vi "Main.vi"(10 "Sub Panel":refnum<vi>, 11 "Module Admin":refnum<class "Delacor_lib_QMH_Module Admin.lvclass">) -> ()   [LabVIEW 2020, in "Acquisition.lvlib"]
doc: "This template is based off of the Queued Message Handler design pattern and the Queued Message Handler project template that ships with LabVIEW.\n\nThe main difference is that the queue is private to this module and communication between modules is performed via Broadcast and Request events.\n\nRequest events are wrapped in public API methods and are handled in the Event Handling Loop (EHL) of this VI. Any module can register for Broadcast events sent by this module. The EHL generates messages based on user interface actions.\n\nThe Message Handling Loop (MHL) processes messages generated by the EHL, or by other messages. The messages are string values, so new messages can be added easily to the Message Cases case structure in the MHL. Each message cluster can also provide an optional value for Message Data, which is a variant that can be converted to whatever message-specific data is required.\n_____\nBased on Delacor QMH Project Template 5.0.0.82."
uses:
  Acquisition.lvlib
  <vilib>/Delacor/Delacor QMH/Libraries/Module Admin_class/Delacor_lib_QMH_Module Admin.lvclass
  Module Data--cluster.ctl
  Stop Helper Loop Argument--cluster.ctl
  Stop Argument--cluster.ctl
  <vilib>/Delacor/Delacor QMH/Libraries/Message Queue_class/Delacor_lib_QMH_Message Queue.lvclass/Delacor_lib_QMH_Message Queue.ctl
  <vilib>/Delacor/Delacor QMH/Libraries/Module Admin_class/Delacor_lib_QMH_Module Admin.lvclass/Delacor_lib_QMH_Module Admin.ctl
  <vilib>/Utility/miscctls.llb/LVPointTypeDef.ctl
  <vilib>/Delacor/Delacor QMH/Libraries/Message Queue_class/Delacor_lib_QMH_Enqueue Message (Single).vi
  <vilib>/Delacor/Delacor QMH/Libraries/Module Admin_class/Delacor_lib_QMH_Get External Launch.vi
  <vilib>/Utility/error.llb/Error Cluster From Error Code.vi
  <vilib>/ErrorRing/Error Ring.xnode
  <vilib>/Delacor/Delacor QMH/Libraries/Message Queue_class/Delacor_lib_QMH_Message Queue.lvclass
  <vilib>/measure/NI_MABase.lvlib
panel:
  out "Waveform Graph":waveform(dbl)(graph)
  out "error out":errorcluster
  out "Status":string
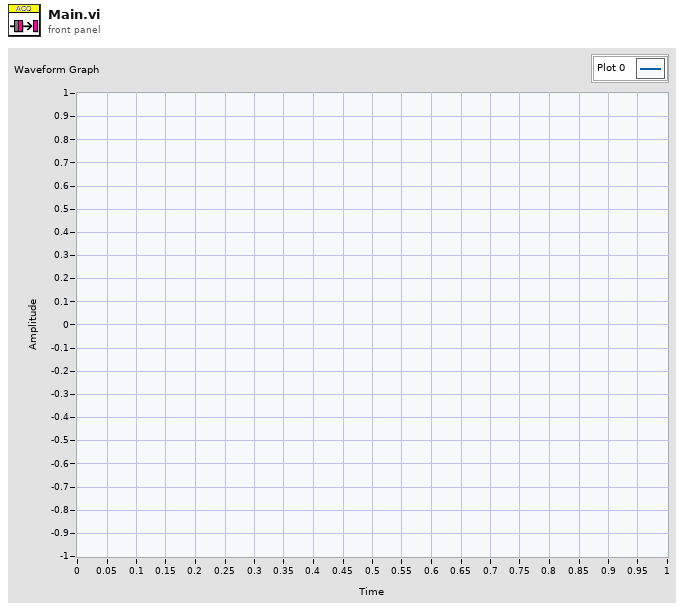
[diagram p1: front panel]
types:
  T1 = typedef "Acquisition.lvlib/Request Events--cluster.ctl" = cluster{"Stop Module":refnum<user-event>, "Show Panel":refnum<user-event>, "Hide Panel":refnum<user-event>, "Get Module Execution Status":refnum<user-event>, "Show Diagram":refnum<user-event>, "Start Helper Loop":refnum<user-event>, "Stop Helper Loop":refnum<user-event>, "Set Acquisition Config":refnum<user-event>}
  T2 = typedef "Acquisition.lvlib/Module Data--cluster.ctl" = cluster{"Status":string}
  T3 = typedef "Acquisition.lvlib/Stop Helper Loop Argument--cluster.ctl" = cluster{"Boolean":bool}
  T4 = enum32{"invalid lock state", "Not Locked", "Locked (No Password)", "Password-protected"}
  T5 = typedef "Acquisition.lvlib/Stop Argument--cluster.ctl" = cluster{"Origin":string, "Exit via Stop Module Req?":bool, "Wait for Module to stop?":bool}
  T6 = typedef "LVPointTypeDef.ctl" = cluster{"Horizontal":i16, "Vertical":i16}
  T7 = enum32{"Invalid", "Standard", "Closed", "Hidden", "Minimized", "Maximized"}
  T8 = enum16{"Sine Wave", "Triangle Wave", "Square Wave", "Sawtooth Wave"}
  T9 = cluster{"sampling info":cluster{"Fs":dbl, "#s":dbl}, "square wave duty cycle (%)":dbl, "frequency":dbl, "amplitude":dbl, "phase":dbl, "signal type":enum16{"Sine Wave", "Triangle Wave", "Square Wave", "Sawtooth Wave"}}
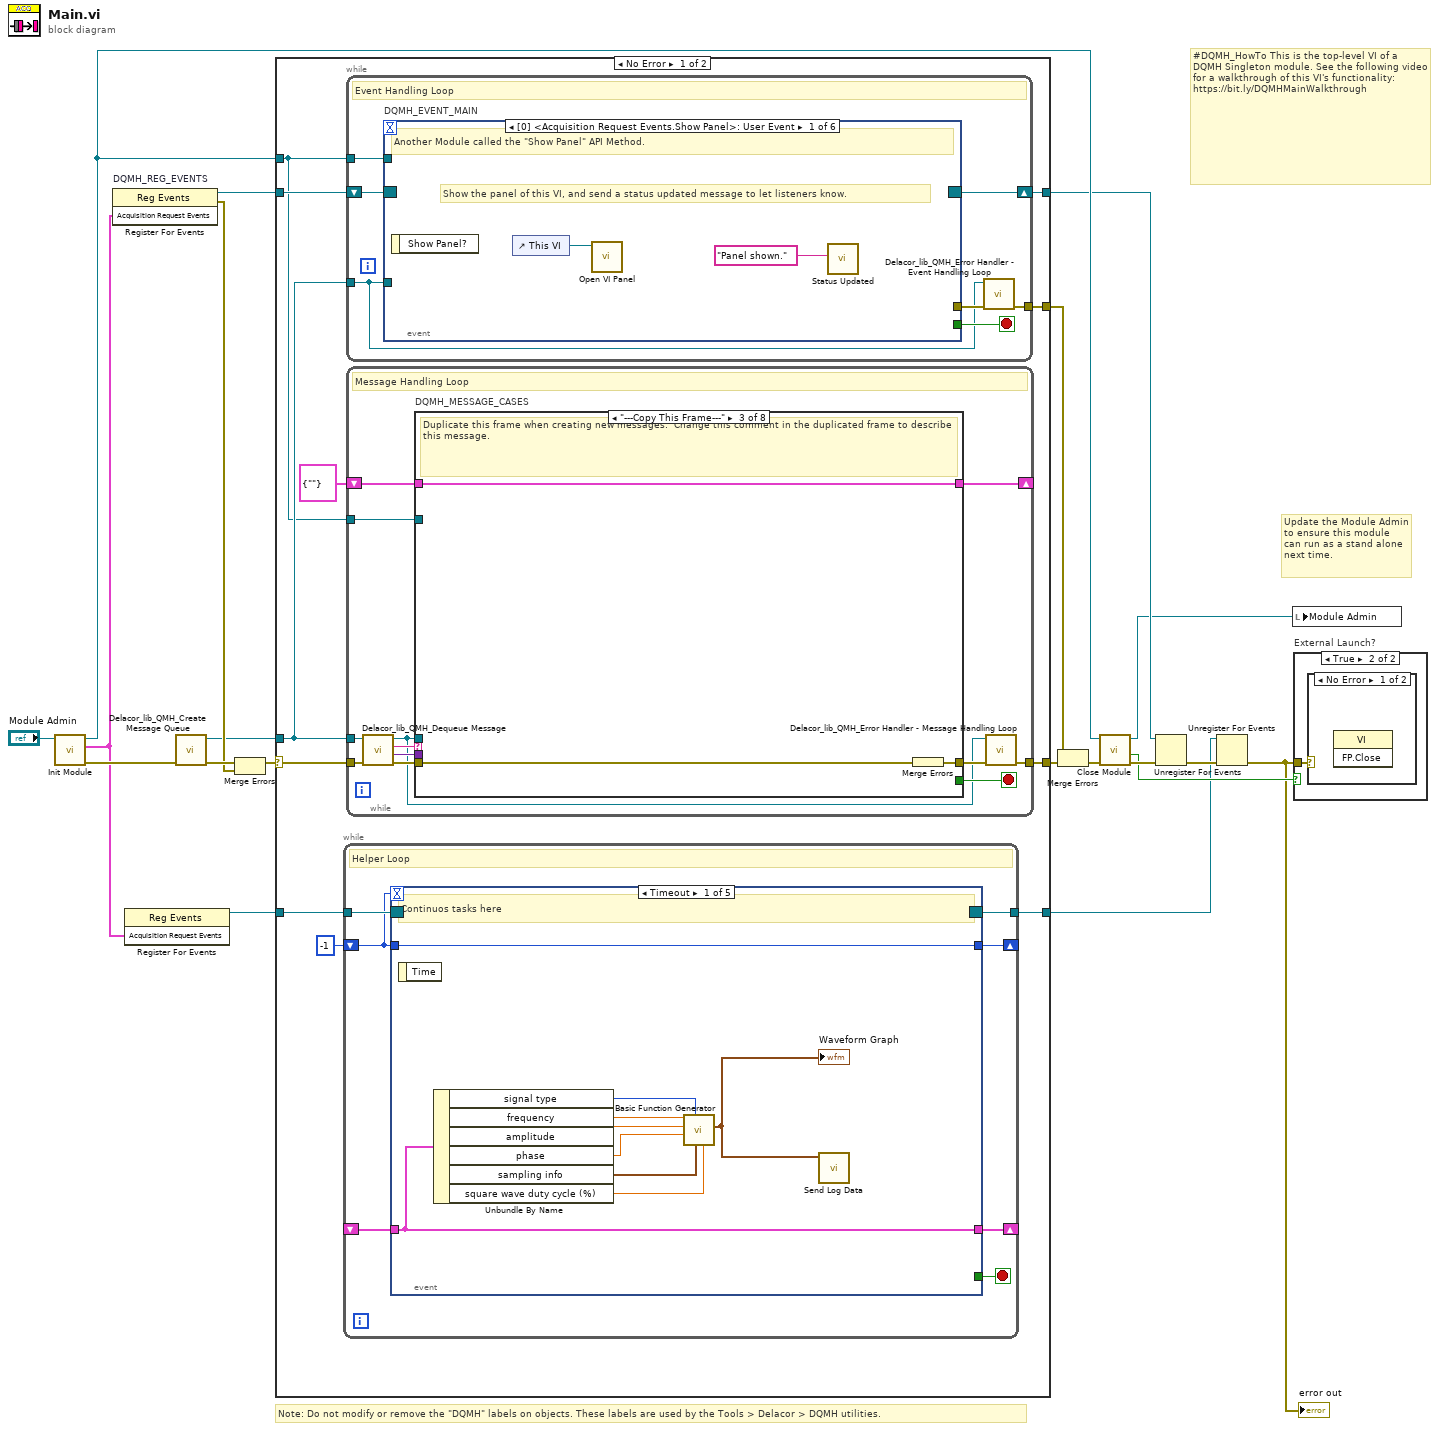
[diagram p0: block diagram]
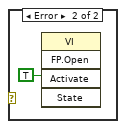
[diagram p3: hidden frame]
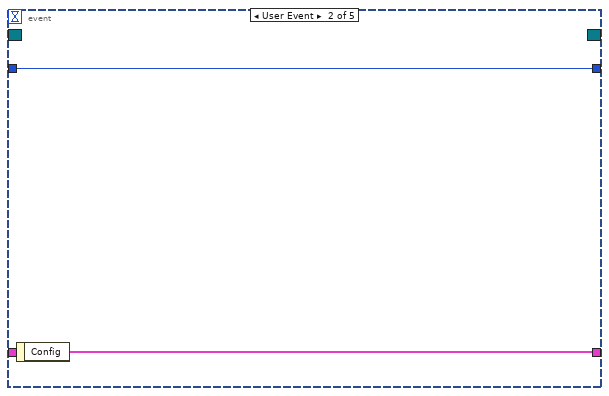
[diagram p4: hidden frame]
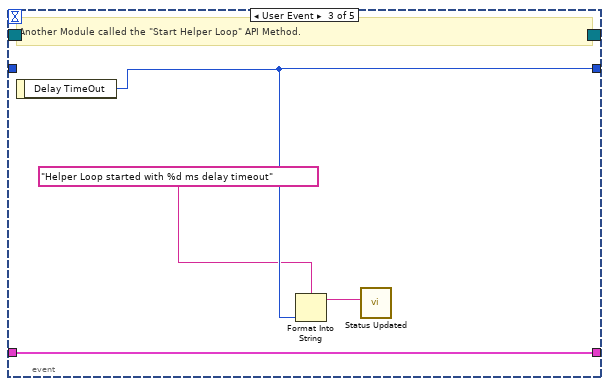
[diagram p5: hidden frame]
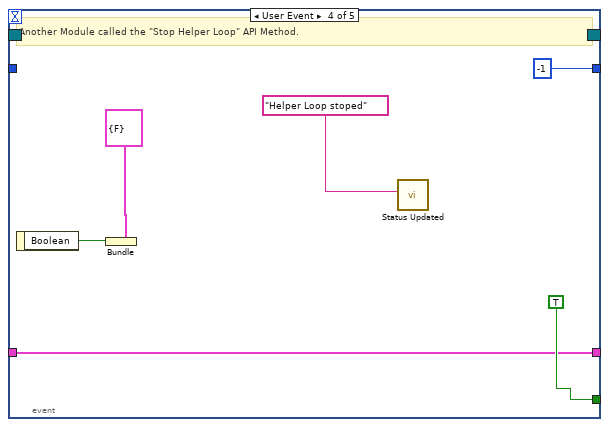
[diagram p6: hidden frame]
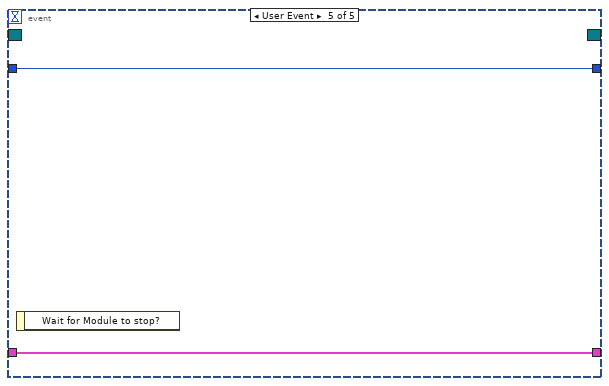
[diagram p7: hidden frame]
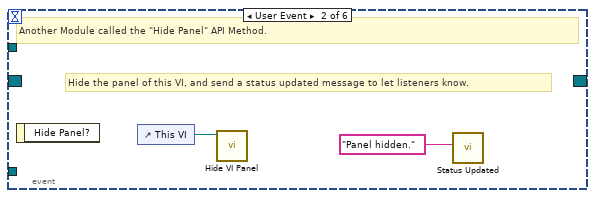
[diagram p8: hidden frame]
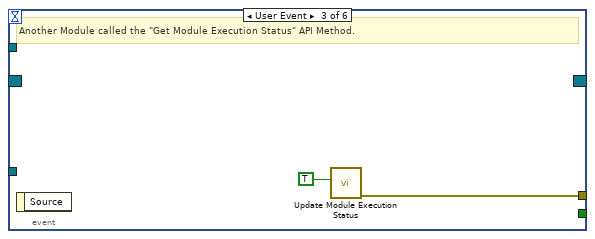
[diagram p9: hidden frame]
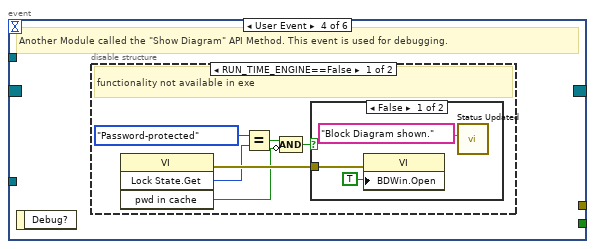
[diagram p10: hidden frame]
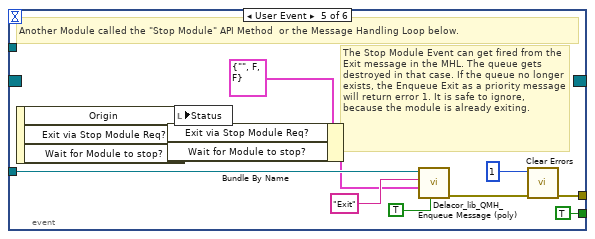
[diagram p13: hidden frame]
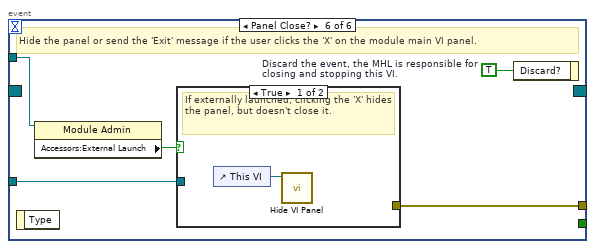
[diagram p14: hidden frame]
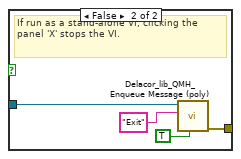
[diagram p15: hidden frame]
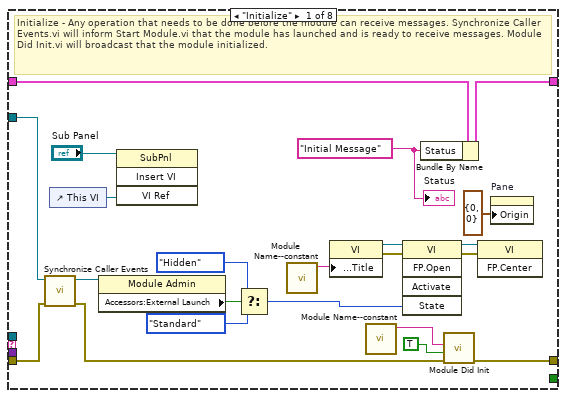
[diagram p16: hidden frame]
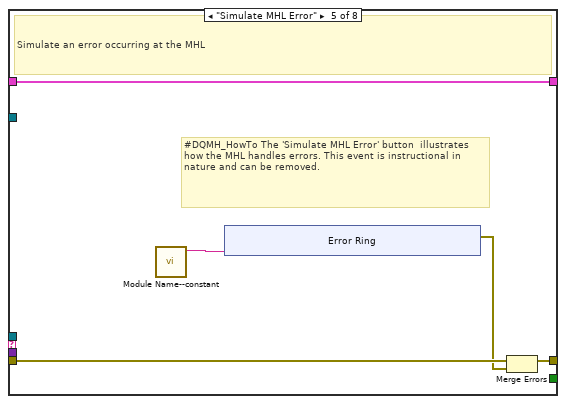
[diagram p19: hidden frame]
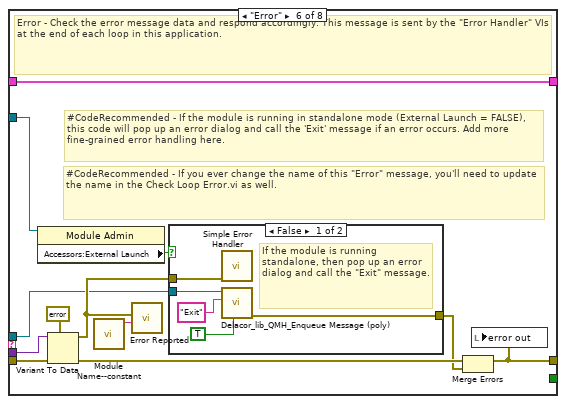
[diagram p20: hidden frame]
diagram:
  # "#DQMH_HowTo This is the top-level VI of a DQMH Singleton module. See the following video for a walkthrough of this VI's functionality: https://bit.ly/DQMHMainWalkthrough"
  # "Note: Do not modify or remove the \"DQMH\" labels on objects. These labels are used by the Tools > Delacor > DQMH utilities."
  # "Update the Module Admin to ensure this module can run as a stand alone next time."
  n1 = call "Init Module.vi"("Singleton Module Admin in"="Module Admin") -> ("error out"=w19:errorcluster, "Acquisition Request Events"=w3:T1, "Singleton Module Admin out"=w11:refnum<class "Delacor_lib_QMH_Module Admin.lvclass">)  [unwired: 8 in]
  n2 = register-events "DQMH_REG_EVENTS"(w3) -> (reference out=w9:refnum<event-registration>, error out=w12:errorcluster)  [unwired: 2 in]
  n3 = register-events(w3) -> (reference out=w4:refnum<event-registration>)  [unwired: 2 in, 1 out]
  n4 = call <vilib>:"Delacor_lib_QMH_Create Message Queue.vi"("error in (no error)"=w19) -> ("error out"=w14:errorcluster, "Message Queue"=w8:refnum<class "Delacor_lib_QMH_Message Queue.lvclass">)  [unwired: 9 in]
  n5 = Merge Errors(w14, w12) -> (w13:errorcluster)
  n6 = case shown="No Error" w13 {
    selector: w13 -> [w29 w207]
    tunnel: [w31 w206] -> w20
    tunnel: [w28 w212] -> w10
    tunnel: w9 -> [w26 w212]
    tunnel: w8 -> [w25 w205]
    tunnel: [w30 _] -> w17
    tunnel: w11 -> [w24 w208]
    tunnel: w4 -> [w23 _]
    tunnel: [w22 _] -> w1
    frame No Error {
      n7 = while {
        tunnel: w23 -> [w38]
        tunnel: [w37] -> w22
        shift-right: [w36] -> _
        shift-left: -1 -> [w35]
        shift-right: [w33] -> _
        shift-left: _ -> [w32]
        stop <- w34 stop-if-true
        # "Helper Loop"
        n8 = event shown="[0] Timeout" {
          selector: w38 -> [_ _ _ _ _]
          dyn-events: [_ _ _ _ _] -> w37
          timeout: w35 -> [_ _ _ _ _]
          tunnel: [w47 w49 w52 -1 w61] -> w36
          tunnel: w35 -> [w47 w49 _ _ w61]
          tunnel: [_ _ _ TRUE _] -> w34
          tunnel: [w46 w48 w50 w54 w60] -> w33
          tunnel: w32 -> [w46 _ w50 w54 w60]
          event Timeout {
            # "Continuos tasks here"
            n9 = event-data() -> ()  [unwired: 1 in, 1 out]
            n10 = Unbundle By Name(w46) -> ("signal type"=w45:T8, "frequency"=w44:dbl, "amplitude"=w43:dbl, "phase"=w42:dbl, "sampling info"=w41:cluster{"Fs":dbl, "#s":dbl}, "square wave duty cycle (%)"=w40:dbl)
            n11 = call <vilib>:"Basic Function Generator.vi"("square wave duty cycle (%)"=w40, "sampling info"=w41, "signal type"=w45, "phase"=w42, "amplitude"=w43, "frequency"=w44) -> ("signal out"=w39:waveform(dbl))  [unwired: 3 in, 2 out]
            "Waveform Graph" <- w39
            n12 = call "Send Log Data.vi"("signal in"=w39) -> ()  [unwired: 11 in]
          }
          event User Event {
            n13 = event-data() -> ("Config"=w48:T9)  [unwired: 1 in]
          }
          event User Event {
            # "Another Module called the \"Start Helper Loop\" API Method."
            n14 = event-data() -> ("Delay TimeOut"=w52:i32)  [unwired: 1 in]
            n15 = Format Into String(format string="Helper Loop started with %d ms delay timeout", w52) -> (resulting string=w53:string)  [unwired: 2 in, 1 out]
            n16 = call "Status Updated.vi"("Status"=w53) -> ()  [unwired: 10 in, 1 out]
          }
          event User Event {
            # "Another Module called the \"Stop Helper Loop\" API Method."
            n17 = event-data() -> ("Boolean"=w58:bool)  [unwired: 1 in]
            n18 = Bundle(cluster=T3 {"Boolean"=FALSE} ("Stop Helper Loop Argument"), "Boolean"=w58) -> ()  [unwired: 1 out]
            n19 = call "Status Updated.vi"("Status"="Helper Loop stoped") -> ()  [unwired: 10 in, 1 out]
          }
          event User Event {
            n20 = event-data() -> ()  [unwired: 1 in, 1 out]
          }
        }
      }
      n21 = while {
        tunnel: w25 -> [w62]
        shift-right: [w65] -> w28
        shift-left: w26 -> [w66]
        tunnel: [w67] -> w30
        tunnel: w24 -> [w63]
        stop <- w64 stop-if-true
        # "Event Handling Loop"
        n22 = event "DQMH_EVENT_MAIN" shown="[0] <Acquisition Request Events.Show Panel>: User Event" {
          selector: w66 -> [_ _ _ _ _ _]
          dyn-events: [_ _ _ _ _ _] -> w65
          timeout: _ -> [_ _ _ _ _ _]
          tunnel: [_ _ _ _ TRUE ("Discard?") _] -> w64
          tunnel: w62 -> [_ _ _ _ w91 w98]
          tunnel: [_ _ w74 _ w94 w100] -> w68
          tunnel: w63 -> [_ _ _ _ _ w97]
          event User Event {
            # "Show the panel of this VI, and send a status updated message to let listeners know."
            # "Another Module called the \"Show Panel\" API Method."
            n23 = event-data() -> ()  [unwired: 1 in, 1 out]
            n24 = control-ref of="This VI"() -> (w70:refnum<vi>)
            n25 = call "Open VI Panel.vi"("VI"=w70) -> ()  [unwired: 10 in, 1 out]
            n26 = call "Status Updated.vi"("Status"="Panel shown." ("format string")) -> ()  [unwired: 10 in, 1 out]
          }
          event User Event {
            # "Hide the panel of this VI, and send a status updated message to let listeners know."
            # "Another Module called the \"Hide Panel\" API Method."
            n27 = event-data() -> ()  [unwired: 1 in, 1 out]
            n28 = control-ref of="This VI"() -> (w72:refnum<vi>)
            n29 = call "Hide VI Panel.vi"("VI"=w72) -> ()  [unwired: 10 in, 1 out]
            n30 = call "Status Updated.vi"("Status"="Panel hidden." ("format string")) -> ()  [unwired: 10 in, 1 out]
          }
          event User Event {
            # "Another Module called the \"Get Module Execution Status\" API Method."
            n31 = event-data() -> ()  [unwired: 1 in, 1 out]
            n32 = call "Update Module Execution Status.vi"("Running?"=TRUE) -> ("error out"=w74:errorcluster)  [unwired: 10 in]
          }
          event User Event {
            # "Another Module called the \"Show Diagram\" API Method. This event is used for debugging."
            n33 = event-data() -> ()  [unwired: 1 in, 1 out]
            n34 = disable-structure shown="RUN_TIME_ENGINE==False" {
              frame condition #0 (active) {
                # "functionality not available in exe"
                n35 = invoke class="VI" method="Lock State.Get"() -> (error out=w80:errorcluster, "Get Lock State"=w79:T4, "pwd in cache"=w76:bool)  [unwired: 4 in, 1 out]
                n36 = Equal?(x=T4."Password-protected", y=w79) -> (x = y?=w77:bool)
                n37 = Compound Arithmetic op=AND(w77, invert w76) -> (w75:bool)
                n38 = case shown="False" w75 {
                  tunnel: w80 -> [w83 _]
                  frame False {
                    n39 = property class="VI"(error in=w83, "BDWin.Open"=TRUE ("Block Diagram Window:Open")) -> ()  [unwired: 1 in, 2 out]
                    n40 = call "Status Updated.vi"("Status"="Block Diagram shown." ("format string")) -> ()  [unwired: 10 in, 1 out]
                  }
                  frame True {
                    # "Password-protected VI, and the password is not in the cache. Do not show the diagram."
                  }
                }
              }
              frame condition #1 {
              }
            }
          }
          event User Event {
            # "The Stop Module Event can get fired from the Exit message in the MHL. The queue gets destroyed in that case. If the queue no longer exists, the Enqueue Exit as a priority message will return error 1. It is safe to ignore, because the module is already exiting."
            # "Another Module called the \"Stop Module\" API Method  or the Message Handling Loop below."
            n41 = event-data() -> ("Origin"=w90:string, "Exit via Stop Module Req?"=w86:bool, "Wait for Module to stop?"=w85:bool)  [unwired: 1 in]
            n42 = Bundle By Name(cluster=T5 {"Origin"="", "Exit via Stop Module Req?"=FALSE, "Wait for Module to stop?"=FALSE} ("Stop Argument"), "Exit via Stop Module Req?"=w86, "Wait for Module to stop?"=w85) -> (w84:T5)
            n43 = local write "Status"(w90) -> ()
            n44 = call-poly <vilib>:"Delacor_lib_QMH_Enqueue Message (poly).vi"("Priority Message? (F)"=TRUE, "Message Data"=w84, "Message"="Exit", "Message Queue in"=w91) -> ("error out"=w95:errorcluster)  [unwired: 6 in, 1 out]
            n45 = call <vilib>:"Clear Errors.vi"("error in (no error)"=w95, "specific error code to clear (0: all)"=1) -> ("error out"=w94:errorcluster)  [unwired: 4 in, 1 out]
          }
          event Panel Close? {
            w99 = TRUE  # Discard the event, the MHL is responsible for closing and stopping this VI.
            # "Hide the panel or send the 'Exit' message if the user clicks the 'X' on the module main VI panel."
            n46 = event-data() -> ()  [unwired: 1 in, 1 out]
            n47 = property class="Module Admin"(reference=w97) -> ("Accessors:External Launch"=w96:bool)  [unwired: 1 in, 2 out]
            n48 = case shown="True" w96 {
              tunnel: w98 -> [_ w104]
              tunnel: [_ w105] -> w100
              frame True {
                # "If externally launched, clicking the 'X' hides the panel, but doesn't close it."
                n49 = control-ref of="This VI"() -> (w101:refnum<vi>)
                n50 = call "Hide VI Panel.vi"("VI"=w101) -> ()  [unwired: 10 in, 1 out]
              }
              frame False {
                # "If run as a stand-alone VI, clicking the panel 'X' stops the VI."
                n51 = call-poly <vilib>:"Delacor_lib_QMH_Enqueue Message (poly).vi"("Priority Message? (F)"=TRUE, "Message"="Exit", "Message Queue in"=w104) -> ("error out"=w105:errorcluster)  [unwired: 7 in, 1 out]
              }
            }
            n52 = event-data("Discard?"=w99) -> ()  [unwired: 1 in, 1 out]
          }
        }
        n53 = call-dynamic "Delacor_lib_QMH_Error Handler - Event Handling Loop.vi"("error in (no error)"=w68, "Message Queue in"=w62) -> ("dup error in"=w67:errorcluster)  [unwired: 8 in, 1 out]
      }
      n54 = while {
        tunnel: w25 -> [w108]
        shift-right: [w112] -> _
        shift-left: T2 {"Status"=""} ("Data Cluster") -> [w113]
        tunnel: w29 -> [w116]
        tunnel: [w114] -> w31
        tunnel: w24 -> [w106]
        stop <- w111 stop-if-true
        # "Message Handling Loop"
        n55 = call-dynamic "Delacor_lib_QMH_Dequeue Message.vi"("error in (no error)"=w116, "Message Queue in"=w108) -> ("error out"=w115:errorcluster, "Message Data"=w109:variant, "Message"=w110:string, "Message Queue out"=w107:refnum<class "Delacor_lib_QMH_Message Queue.lvclass">)  [unwired: 6 in]
        n56 = case "DQMH_MESSAGE_CASES" shown="\"---Copy This Frame---\"" w110 {
          selector: w110 -> [_ _ _ _ _ _ _ w192]
          tunnel: w107 -> [_ _ _ _ _ w162 w184 _]
          tunnel: w115 -> [w137 w141 w144 w146 w151 w169 w190 w194]
          tunnel: [w135 w141 w143 w146 w150 w165 w187 w195] -> w117
          tunnel: w113 -> [w126 w140 w142 w145 w148 w164 w183 w193]
          tunnel: [w125 w140 w142 w145 w148 w164 w183 w193] -> w112
          tunnel: [_ _ _ _ _ _ w182 _] -> w111
          tunnel: w109 -> [_ _ _ _ _ w163 w181 _]
          tunnel: w106 -> [w127 _ _ _ _ w161 w176 _]
          frame "Initialize" {
            w120 = "Initial Message" ("Initial Message")
            # "Initialize - Any operation that needs to be done before the module can receive messages. Synchronize Caller Events.vi will inform Start Module.vi that the module has launched and is ready to receive messages. Module Did Init.vi will broadcast that the module initialized."
            n57 = call "Synchronize Caller Events.vi"("error in (no error)"=w137, "Singleton Module Admin in"=w127) -> ("error out"=w136:errorcluster, "Singleton Module Admin out"=w122:refnum<class "Delacor_lib_QMH_Module Admin.lvclass">)  [unwired: 8 in]
            n58 = control-ref of="This VI"() -> (w118:refnum<vi>)
            n59 = property class="Module Admin"(reference=w122) -> ("Accessors:External Launch"=w131:bool)  [unwired: 1 in, 2 out]
            n60 = invoke class="SubPnl" method="Insert VI"(reference="Sub Panel", "VI Ref"=w118) -> ()  [unwired: 2 in, 4 out]
            n61 = Select(t=T7."Hidden" ("State"), s=w131, f=T7."Standard" ("State")) -> (s? t:f=w128:T7)
            n62 = call "Module Name--constant.vi"() -> ("Module Name"=w134:string)  [unwired: 11 in]
            n63 = property class="VI"("Front Panel.Title"=w134) -> (reference out=w133:refnum<vi>, error out=w139:errorcluster)  [unwired: 2 in]
            n64 = call "Module Name--constant.vi"() -> ("Module Name"=w123:string)  [unwired: 11 in]
            n65 = invoke class="VI" method="FP.Open"(reference=w133, error in=w139, "State"=w128) -> (reference out=w132:refnum<vi>, error out=w138:errorcluster)  [unwired: 2 in, 3 out]
            n66 = Bundle By Name(cluster=w126, "Status"=w120) -> (w125:T2)
            n67 = call "Module Did Init.vi"("error in (no error)"=w136, "Initialized?"=TRUE, "Origin"=w123) -> ("error out"=w135:errorcluster)  [unwired: 8 in]
            n68 = invoke class="VI" method="FP.Center"(reference=w132, error in=w138) -> ()  [unwired: 1 in, 3 out]
            n69 = property on="Pane" class="Pane"("Origin"=T6 {"Horizontal"=0, "Vertical"=0}) -> ()  [unwired: 2 in, 2 out]
            "Status" <- w120
          }
          frame "--- Module Specific ---" {
            # "Separator -- The following cases handle messages specific to this Module."
          }
          frame "---Copy This Frame---" {
            # "Duplicate this frame when creating new messages.  Change this comment in the duplicated frame to describe this message."
            n70 = Merge Errors(w144) -> (w143:errorcluster)
          }
          frame "--- Exit and Error Handling---" {
            # "Separator - The following cases handle errors and exit messages."
          }
          frame "Simulate MHL Error" {
            # "#DQMH_HowTo The 'Simulate MHL Error' button  illustrates how the MHL handles errors. This event is instructional in nature and can be removed."
            # "Simulate an error occurring at the MHL"
            n71 = call "Module Name--constant.vi"() -> ("Module Name"=w147:string)  [unwired: 11 in]
            n72 = xnode "Error Ring"("parameter 0"=w147) -> ("error out"=w149:errorcluster)
            n73 = Merge Errors(w151, w149) -> (w150:errorcluster)
          }
          frame "Error" {
            # "#CodeRecommended - If you ever change the name of this \"Error\" message, you'll need to update the name in the Check Loop Error.vi as well."
            # "#CodeRecommended - If the module is running in standalone mode (External Launch = FALSE), this code will pop up an error dialog and call the 'Exit' message if an error occurs. Add more fine-grained error handling here."
            # "Error - Check the error message data and respond accordingly. This message is sent by the \"Error Handler\" VIs at the end of each loop in this application."
            n74 = property class="Module Admin"(reference=w161) -> ("Accessors:External Launch"=w160:bool)  [unwired: 1 in, 2 out]
            n75 = Variant To Data(error in=w169, type=errorcluster {"status"=FALSE, "code"=0, "source"=""} ("error constant"), Variant=w163) -> (data=w170:errorcluster, error out=w167:errorcluster)
            n76 = call "Module Name--constant.vi"() -> ("Module Name"=w159:string)  [unwired: 11 in]
            n77 = call "Error Reported.vi"("Additional Information"=w159, "Error"=w170) -> ()  [unwired: 9 in, 1 out]
            n78 = case shown="False" w160 {
              tunnel: [w175 _] -> w166
              tunnel: w162 -> [w173 _]
              tunnel: w170 -> [w174 _]
              frame False {
                # "If the module is running standalone, then pop up an error dialog and call the \"Exit\" message."
                n79 = call <vilib>:"Simple Error Handler.vi"("error in (no error)"=w174) -> ()  [unwired: 4 in, 5 out]
                n80 = call-poly <vilib>:"Delacor_lib_QMH_Enqueue Message (poly).vi"("Priority Message? (F)"=TRUE, "Message"="Exit", "Message Queue in"=w173) -> ("error out"=w175:errorcluster)  [unwired: 7 in, 1 out]
              }
              frame True {
                # "If the module was launched externally, calling the Error Reported broadcast VI is the only action performed by the \"Error\" message. The module's caller can then process the error appropriately."
              }
            }
            n81 = Merge Errors(w167, w166) -> (w165:errorcluster)
            n82 = local write "error out"(w165) -> ()
          }
          frame "Exit" {
            w180 = 91  # 91: not all Exit messages will have an argument
            w182 = TRUE  # Stop the VI
            # "Release the message queue reference"
            # "#CodeNeeded - Add any required cleanup code here"
            # "Exit - Exit the application."
            n83 = Variant To Data(error in=w190, type=T5 {"Origin"="", "Exit via Stop Module Req?"=FALSE, "Wait for Module to stop?"=FALSE} ("Stop Argument"), Variant=w181) -> (data=w178:T5, error out=w186:errorcluster)
            n84 = call <vilib>:"Clear Errors.vi"("error in (no error)"=w186, "specific error code to clear (0: all)"=w180) -> ("error out"=w189:errorcluster)  [unwired: 4 in, 1 out]
            n85 = control-ref of="This VI"() -> (w177:refnum<vi>)
            n86 = call-dynamic "Delacor_lib_QMH_Release Message Queue.vi"("error in (no error)"=w189, "Message Queue"=w184) -> ("error out"=w188:errorcluster)  [unwired: 9 in]
            n87 = call "Handle Exit.vi"("Stop Argument"=w178, "Admin in"=w176, "VI reference"=w177) -> ("error out"=w185:errorcluster)  [unwired: 7 in, 1 out]
            n88 = Merge Errors(w188, w185) -> (w187:errorcluster)
          }
          frame Default {
            # "'Default' case only runs if there is a message that isn't defined in any of the other cases.  Output a programming error."
            n89 = call "Module Name--constant.vi"() -> ("Module Name"=w191:string)  [unwired: 11 in]
            n90 = xnode "Error Ring"("parameter 0"=w192, "parameter 1"=w191) -> ("error out"=w196:errorcluster)
            n91 = Merge Errors(w194, w196) -> (w195:errorcluster)
          }
        }
        n92 = call-dynamic "Delacor_lib_QMH_Error Handler - Message Handling Loop.vi"("error in (no error)"=w117, "Message Queue in"=w107) -> ("dup error in"=w114:errorcluster)  [unwired: 8 in, 1 out]
      }
    }
    frame Error {
      # "Synchronize Caller Events.vi will inform Start Module.vi that the module has launched and will let the code calling Start Module.vi register for broadcasts and would permit the caller receive the broadcast that an error occurred at launch time."
      n93 = call-dynamic "Delacor_lib_QMH_Release Message Queue.vi"("error in (no error)"=w207, "Message Queue"=w205) -> ("error out"=w206:errorcluster)  [unwired: 9 in]
      n94 = call "Synchronize Caller Events.vi"("Singleton Module Admin in"=w208) -> ("error out"=w213:errorcluster)  [unwired: 9 in, 1 out]
      n95 = call "Module Name--constant.vi"() -> ("Module Name"=w211:string)  [unwired: 11 in]
      n96 = Format Into String(format string="An error occurred during initialization. %s is no longer running.", w211) -> (resulting string=w209:string)  [unwired: 2 in, 1 out]
      n97 = Merge Errors(w206, w213) -> (w214:errorcluster)
      n98 = call "Error Reported.vi"("Additional Information"=w209, "Error"=w214) -> ()  [unwired: 9 in, 1 out]
    }
  }
  n99 = Merge Errors(w17, w20) -> (w16:errorcluster)
  n100 = call "Close Module.vi"("error in (no error)"=w16, "Module Admin in"=w11) -> ("error out"=w18:errorcluster, "External Launch"=w5:bool, "Module Admin out"=w6:refnum<class "Delacor_lib_QMH_Module Admin.lvclass">)  [unwired: 7 in]
  n101 = Unregister For Events(event registration refnum=w10, error in=w18) -> (error out=w15:errorcluster)
  n102 = Unregister For Events(event registration refnum=w1, error in=w15) -> (error out=w2:errorcluster)
  "error out" <- w2
  n103 = local write "Module Admin"(w6) -> ()
  n104 = case "External Launch?" shown="True" w5 {
    tunnel: w2 -> [_ w215]
    frame False {
    }
    frame True {
      n105 = case shown="No Error" w215 {
        frame No Error {
          n106 = invoke class="VI" method="FP.Close"() -> ()  [unwired: 3 in, 3 out]
        }
        frame Error {
          n107 = invoke class="VI" method="FP.Open"("Activate"=TRUE ("Activate?")) -> ()  [unwired: 4 in, 5 out]
        }
      }
    }
  }
